vi "Periodic Tasks.vi"(8 "error in":errorcluster) -> ()   [LabVIEW 2017]
doc: "This VI runs in parallel to other tasks. It can contain as many user-defined periodic loops as you need. These can carry out PID or other sorts of timed response."
uses:
  <vilib>/Rock Robotics/WPI/ThirdParty/Phoenix-LabVIEW/Motor Controller/Controls/CTRE_Phoenix_MotorControl_ControlMode.ctl
  <vilib>/Rock Robotics/WPI/ThirdParty/Phoenix-LabVIEW/Motor Controller/Controls/CTRE_Phoenix_MotorControl_LimitSwitchNormal.ctl
  <vilib>/Rock Robotics/WPI/ThirdParty/Phoenix-LabVIEW/Motor Controller/Controls/CTRE_Phoenix_MotorControl_LimitSwitchSource.ctl
  <vilib>/Rock Robotics/WPI/ThirdParty/Phoenix-LabVIEW/Motor Controller/Controls/CTRE_Phoenix_MotorControl_LimitSwitchSource_Local.ctl
  <vilib>/Rock Robotics/WPI/ThirdParty/Phoenix-LabVIEW/Controls/CTRE_Phoenix_Params.ctl
  <vilib>/Rock Robotics/WPI/Utilities/WPI_GetSetVariantRefNum.vi
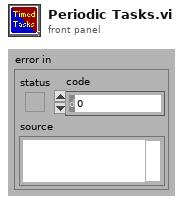
[diagram p1: front panel]
types:
  T1 = typedef "CTRE_CANifier_DeviceRef.ctl" = cluster{"DeviceStatus":errorcluster, "Device Number":u8, "Handle":u64, "UsageFrame":u32, "Library Path":path}
  T2 = typedef "WPI_MotorControlDeviceRef.ctl" = cluster{"DeviceStatus":errorcluster, "Type":T3, "PWM":cluster{"PWM Channel":T4, "DeadBand":T5}, "CAN":cluster{"Device Number":u8, "SetOutput VI Ref":variant, "GetOutput VI Ref":variant, "Enable VI Ref":variant, "Disable VI Ref":variant, "Data":variant}, "Invert":bool, "DIO PWM":cluster{"PWM \"Enable\" Channel":T4, "DIOChannel":T6, "PWM Rate":dbl}}
  T3 = typedef "WPI_MotorControlType.ctl" = enum16{"PWM", "CAN", "DIO PWM"}
  T4 = typedef "FPGA_DIOPWMChannel.ctl" = enum8{"PWM 0", "PWM 1", "PWM 2", "PWM 3", "PWM 4", "PWM 5", "PWM 6", "PWM 7", "PWM 8", "PWM 9", "PWM MXP 0", "PWM MXP 1", "PWM MXP 2", "PWM MXP 3", "PWM MXP 4", "PWM MXP 5", "PWM MXP 6", "PWM MXP 7", "PWM MXP 8", "PWM MXP 9", "Invalid"}
  T5 = typedef "WPI_PWMDeadband.ctl" = cluster{"Name":string, "maxPositivePwm":i32, "minPositivePwm":i32, "centerPwm":i32, "maxNegativePwm":i32, "minNegativePwm":i32, "angularRange":u16}
  T6 = typedef "FPGA_DIOChannel.ctl" = enum8{"DIO 0", "DIO 1", "DIO 2", "DIO 3", "DIO 4", "DIO 5", "DIO 6", "DIO 7", "DIO 8", "DIO 9", "DIO MXP 0", "DIO MXP 1", "DIO MXP 2", "DIO MXP 3", "DIO MXP 4", "DIO MXP 5", "DIO MXP 6", "DIO MXP 7", "DIO MXP 8", "DIO MXP 9", "DIO MXP 10", "DIO MXP 11", "DIO MXP 12", "DIO MXP 13", "DIO MXP 14", "DIO MXP 15", "SPI Port CS1", "SPI Port CS2", "SPI Port CS3", "SPI Port MISO", "SPI Port MOSI", "Invalid"}
  T7 = typedef "WPI_JoystickDevRef.ctl" = cluster{"Device":T8}
  T8 = typedef "WPI_JoystickDeviceEnum.ctl" = enum16{"USB 0", "USB 1", "USB 2", "USB 3", "USB 4", "USB 5"}
  T9 = typedef "CTRE_Phoenix_MotorControl_ControlMode.ctl" = u16
  T10 = typedef "CTRE_Phoenix_MotorControl_LimitSwitchSource.ctl" = u16
  T11 = typedef "CTRE_Phoenix_MotorControl_LimitSwitchNormal.ctl" = enum16{"Normally Open", "Normally Closed", "Disabled"}
  T12 = typedef "CTRE_Phoenix_MotorControl_LimitSwitchSource_Local.ctl" = enum16{"Feedback Connector", "Remote Talon SRX", "Remote CANifier", "Deactivated"}
  T13 = typedef "CTRE_Phoenix_Params.ctl" = u16
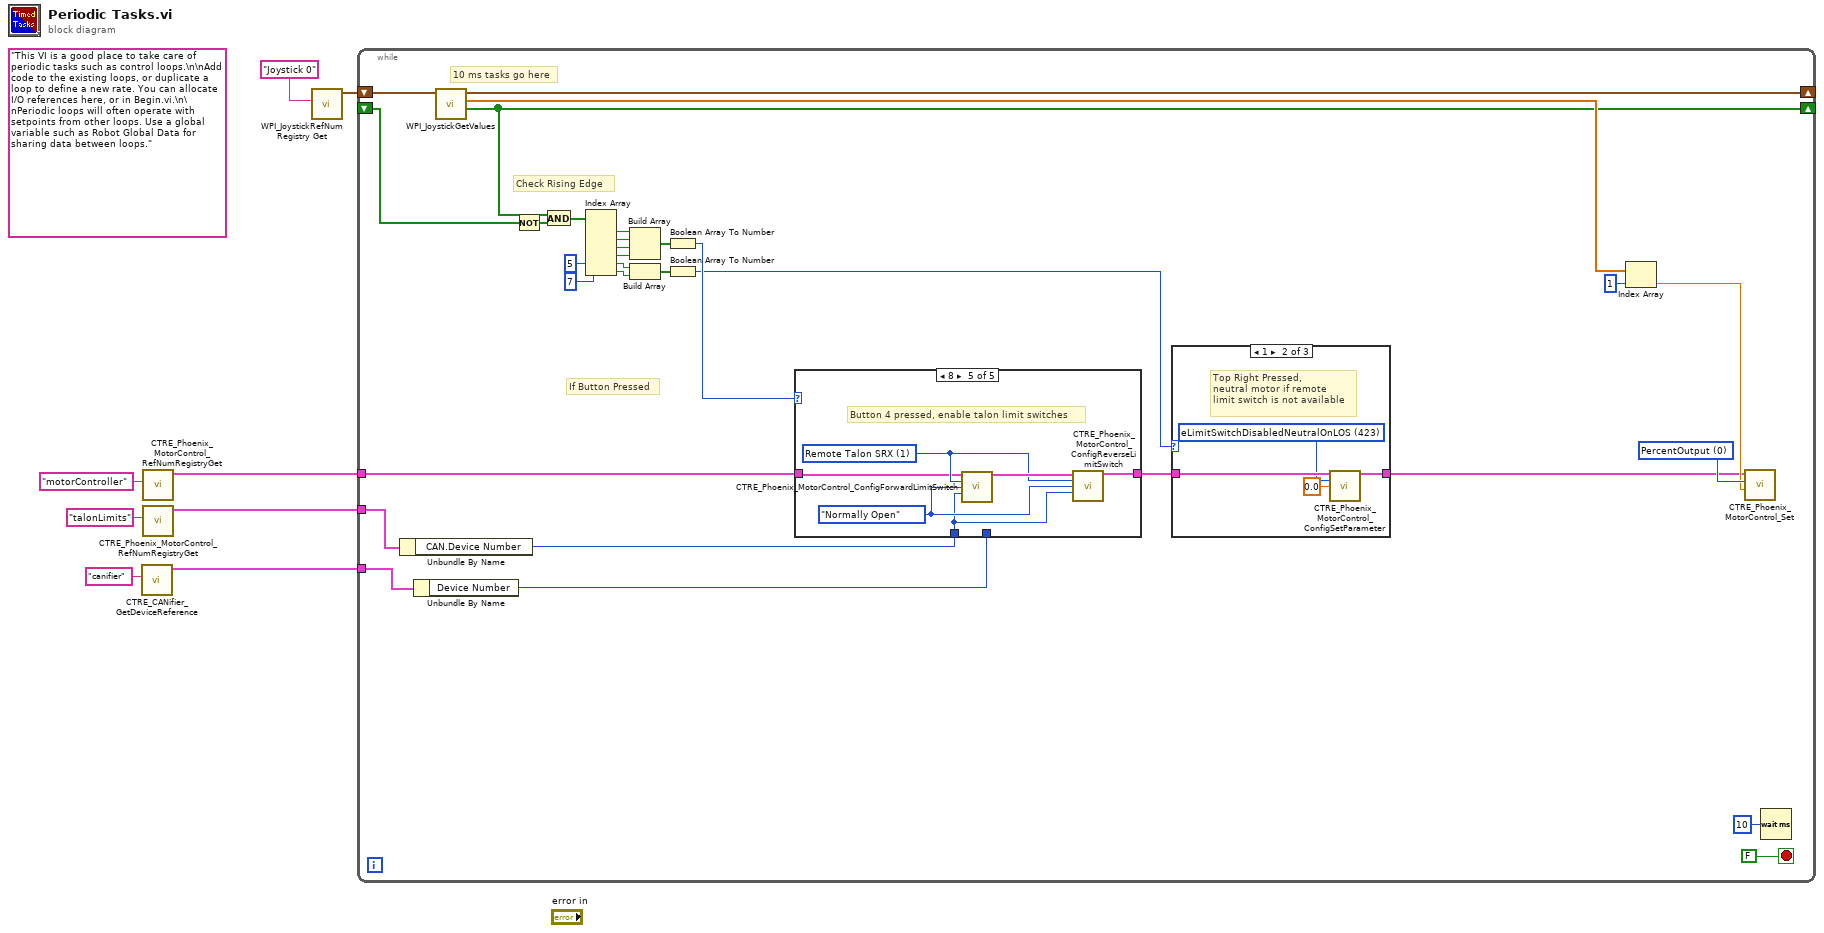
[diagram p0: block diagram]
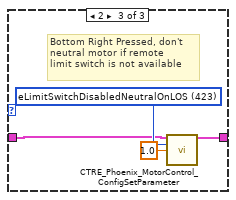
[diagram p3: hidden frame]
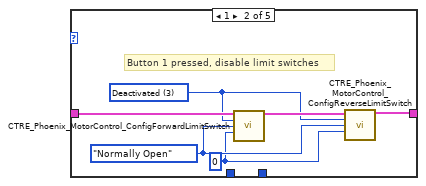
[diagram p5: hidden frame]
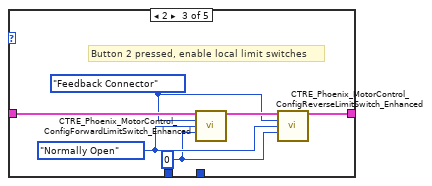
[diagram p6: hidden frame]
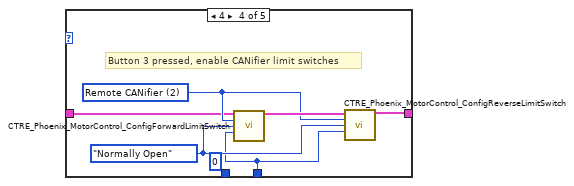
[diagram p7: hidden frame]
diagram:
  (unwired) "This VI is a good place to take care of periodic tasks such as control loops.\n\nAdd code to the existing loops, or duplicate a loop to define a new rate. You can allocate I/O references here, or in Begin.vi.\n\nPeriodic loops will often operate with setpoints from other loops. Use a global variable such as Robot Global Data for sharing data between loops."
  n1 = call <vilib>:"CTRE_CANifier_GetDeviceReference.vi"("refnum name"="canifier") -> ("CANifierDevRef"=w3:T1)  [unwired: 9 in, 1 out]
  n2 = call <vilib>:"CTRE_Phoenix_MotorControl_RefNumRegistryGet.vi"("refnum name"="motorController") -> ("PhoenixMotorControlDevRef"=w1:T2)  [unwired: 9 in, 1 out]
  n3 = call <vilib>:"CTRE_Phoenix_MotorControl_RefNumRegistryGet.vi"("refnum name"="talonLimits") -> ("PhoenixMotorControlDevRef"=w2:T2)  [unwired: 9 in, 1 out]
  n4 = call <vilib>:"WPI_JoystickRefNum Registry Get.vi"("refnum name"="Joystick 0") -> ("JoystickDevRef"=w7:T7)  [unwired: 1 in, 9 out]
  n5 = while {
    shift-right: [w35] -> _
    shift-left: w7 -> [w36]
    tunnel: w3 -> [w23]
    tunnel: w2 -> [w24]
    tunnel: w1 -> [w25]
    shift-right: [w30] -> _
    shift-left: _ -> [w31]
    stop <- FALSE stop-if-true
    w37 = T9 0 items=["PercentOutput"=0, "Position"=1, "Velocity"=2, "Current"=3, "Follower"=5, "MotionProfile"=6, "MotionMagic"=7, "MotionMagicArc"=8, "MotionProfileArc"=10, "Disabled"=15] ("Control Mode")
    # "If Button Pressed"
    # "Check Rising Edge"
    # "10 ms tasks go here"
    n6 = Unbundle By Name(w24) -> ("CAN.Device Number"=w16:u8)
    n7 = Unbundle By Name(w23) -> ("Device Number"=w15:u8)
    n8 = call <vilib>:"WPI_JoystickGetValues.vi"("JoystickDevRef"=w36) -> ("Buttons"=w30:bool[], "Axes"=w34:dbl[], "JoystickDevRef"=w35:T7)  [unwired: 6 in, 2 out]
    n9 = Not(x=w31) -> (.not. x?=w29:bool[])
    n10 = And(x=w30, y=w29) -> (x .and. y?=w26:bool[])
    n11 = Index Array(array=w26, index #5=5 ("index"), index #6=7 ("index")) -> (element #1=w22:bool, element #2=w19:bool, element #3=w20:bool, element #4=w21:bool, element #5=w14:bool, element #6=w13:bool)  [unwired: 4 in]
    n12 = Build Array(w22, w19, w20, w21) -> (w18:bool[])
    n13 = Build Array(w14, w13) -> (w12:bool[])
    n14 = Boolean Array To Number(Boolean array=w18) -> (number=w17:u32)
    n15 = Boolean Array To Number(Boolean array=w12) -> (number=w11:u32)
    n16 = case shown="8" w17 {
      tunnel: w25 -> [w49 w55 w59 w63 w69]
      tunnel: [w49 w53 w60 w62 w70] -> w9
      tunnel: w16 -> [_ _ _ _ w68]
      tunnel: w15 -> [_ _ _ w64 _]
      frame 0, Default {
        # "Nothing pressed"
      }
      frame 1 {
        w52 = T10 3 items=["Remote Talon SRX"=1, "Remote CANifier"=2, "Deactivated"=3] ("LimitSwitchSource")
        w50 = 0 ("deviceID")
        w51 = CTRE_Phoenix_MotorControl_LimitSwitchNormal."Normally Open" ("NormallyOpenOrClosed")
        # "Button 1 pressed, disable limit switches"
        n17 = call <vilib>:"CTRE_Phoenix_MotorControl_ConfigForwardLimitSwitch.vi"("PhoenixMotorControlDevRef"=w55, "LimitSwitchSource"=w52, "NormallyOpenOrClosed"=w51, "deviceID"=w50) -> ("PhoenixMotorControlDevRef"=w54:T2)  [unwired: 10 in, 1 out]
        n18 = call <vilib>:"CTRE_Phoenix_MotorControl_ConfigReverseLimitSwitch.vi"("PhoenixMotorControlDevRef"=w54, "LimitSwitchSource"=w52, "NormallyOpenOrClosed"=w51, "deviceID"=w50) -> ("PhoenixMotorControlDevRef"=w53:T2)  [unwired: 10 in, 1 out]
      }
      frame 2 {
        w56 = 0 ("deviceID")
        w57 = CTRE_Phoenix_MotorControl_LimitSwitchNormal."Normally Open" ("NormallyOpenOrClosed")
        w58 = CTRE_Phoenix_MotorControl_LimitSwitchSource_Local."Feedback Connector" ("Limit Switch Source")
        # "Button 2 pressed, enable local limit switches"
        n19 = call <vilib>:"CTRE_Phoenix_MotorControl_ConfigForwardLimitSwitch_Enhanced.vi"("PhoenixMotorControlDevRef"=w59, "Limit Switch Source"=w58, "NormallyOpenOrClosed"=w57, "deviceID"=w56) -> ("PhoenixMotorControlDevRef"=w61:T2)  [unwired: 10 in, 1 out]
        n20 = call <vilib>:"CTRE_Phoenix_MotorControl_ConfigReverseLimitSwitch_Enhanced.vi"("PhoenixMotorControlDevRef"=w61, "Limit Switch Source"=w58, "NormallyOpenOrClosed"=w57, "deviceID"=w56) -> ("PhoenixMotorControlDevRef"=w60:T2)  [unwired: 10 in, 1 out]
      }
      frame 4 {
        w66 = T10 2 items=["Remote Talon SRX"=1, "Remote CANifier"=2, "Deactivated"=3] ("LimitSwitchSource")
        (unwired) 0 ("deviceID")
        w65 = CTRE_Phoenix_MotorControl_LimitSwitchNormal."Normally Open" ("NormallyOpenOrClosed")
        # "Button 3 pressed, enable CANifier limit switches"
        n21 = call <vilib>:"CTRE_Phoenix_MotorControl_ConfigForwardLimitSwitch.vi"("PhoenixMotorControlDevRef"=w63, "LimitSwitchSource"=w66, "NormallyOpenOrClosed"=w65, "deviceID"=w64) -> ("PhoenixMotorControlDevRef"=w67:T2)  [unwired: 10 in, 1 out]
        n22 = call <vilib>:"CTRE_Phoenix_MotorControl_ConfigReverseLimitSwitch.vi"("PhoenixMotorControlDevRef"=w67, "LimitSwitchSource"=w66, "NormallyOpenOrClosed"=w65, "deviceID"=w64) -> ("PhoenixMotorControlDevRef"=w62:T2)  [unwired: 10 in, 1 out]
      }
      frame 8 {
        w72 = T10 1 items=["Remote Talon SRX"=1, "Remote CANifier"=2, "Deactivated"=3] ("LimitSwitchSource")
        w71 = CTRE_Phoenix_MotorControl_LimitSwitchNormal."Normally Open" ("NormallyOpenOrClosed")
        # "Button 4 pressed, enable talon limit switches"
        n23 = call <vilib>:"CTRE_Phoenix_MotorControl_ConfigForwardLimitSwitch.vi"("PhoenixMotorControlDevRef"=w69, "LimitSwitchSource"=w72, "NormallyOpenOrClosed"=w71, "deviceID"=w68) -> ("PhoenixMotorControlDevRef"=w73:T2)  [unwired: 10 in, 1 out]
        n24 = call <vilib>:"CTRE_Phoenix_MotorControl_ConfigReverseLimitSwitch.vi"("PhoenixMotorControlDevRef"=w73, "LimitSwitchSource"=w72, "NormallyOpenOrClosed"=w71, "deviceID"=w68) -> ("PhoenixMotorControlDevRef"=w70:T2)  [unwired: 10 in, 1 out]
      }
    }
    n25 = case shown="1" w11 {
      tunnel: [w40 w44 w46] -> w10
      tunnel: w9 -> [w40 w43 w45]
      frame 0, Default {
      }
      frame 1 {
        w42 = T13 423 items=["eOnBoot_BrakeMode"=31, "eQuadFilterEn"=91, "eQuadIdxPolarity"=108, "eClearPositionOnIdx"=100, "eMotionProfileHasUnderrunErr"=119, "eMotionProfileTrajectoryPointDurationMs"=120, "eClearPosOnLimitF"=144, "eClearPosOnLimitR"=145, "eStatusFramePeriod"=300, "eOpenLoopRamp"=301, "eClosedLoopRamp"=302, "eNeutralDeadband"=303, "ePeakPosOutput"=305, "eNominalPosOutput"=306, "ePeakNegOutput"=307, "eNominalNegOutput"=308, "eProfileParamSlot_P"=310, "eProfileParamSlot_I"=311, "eProfileParamSlot_D"=312, "eProfileParamSlot_F"=313, "eProfileParamSlot_IZone"=314, "eProfileParamSlot_AllowableErr"=315, "eProfileParamSlot_MaxIAccum"=316, "eClearPositionOnLimitF"=320, "eClearPositionOnLimitR"=321, "eClearPositionOnQuadIdx"=322, "eSampleVelocityPeriod"=325, "eSampleVelocityWindow"=326, "eFeedbackSensorType"=330, "eSelectedSensorPosition"=331, "eFeedbackNotContinuous"=332, "eRemoteSensorSource"=333, "eRemoteSensorDeviceID"=334, "eSensorTerm"=335, "eRemoteSensorClosedLoopDisableNeutralOnLOS"=336, "eForwardSoftLimitThreshold"=340, "eReverseSoftLimitThreshold"=341, "eForwardSoftLimitEnable"=342, "eReverseSoftLimitEnable"=343, "eNominalBatteryVoltage"=350, "eBatterVoltageFilterSize"=351, "eContinuousCurrentLimitAmps"=360, "eContinuousCurrentLimitMs"=361, "ePeakCurrentLimitAmps"=362, "eClosedLoopIAccum"=370, "eCustomParam"=380, "eStickyFaults"=390, "eAnalogPosition"=400, "eQuadraturePosition"=401, "ePulseWidthPosition"=402, "eMotMag_Accel"=410, "eMotMag_VelCruise"=411, "eLimitSwitchSource"=421, "eLimitSwitchNormClosedAndDis"=422, "eLimitSwitchDisabledNeutralOnLOS"=423, "eLimitSwitchRemoteDevID"=424] ("Parameter")
        # "Top Right Pressed,\nneutral motor if remote\nlimit switch is not available"
        n26 = call <vilib>:"CTRE_Phoenix_MotorControl_ConfigSetParameter.vi"("PhoenixMotorControlDevRef"=w43, "Parameter"=w42, "value"=0.0) -> ("PhoenixMotorControlDevRef"=w44:T2)  [unwired: 11 in, 1 out]
      }
      frame 2 {
        w48 = T13 423 items=["eOnBoot_BrakeMode"=31, "eQuadFilterEn"=91, "eQuadIdxPolarity"=108, "eClearPositionOnIdx"=100, "eMotionProfileHasUnderrunErr"=119, "eMotionProfileTrajectoryPointDurationMs"=120, "eClearPosOnLimitF"=144, "eClearPosOnLimitR"=145, "eStatusFramePeriod"=300, "eOpenLoopRamp"=301, "eClosedLoopRamp"=302, "eNeutralDeadband"=303, "ePeakPosOutput"=305, "eNominalPosOutput"=306, "ePeakNegOutput"=307, "eNominalNegOutput"=308, "eProfileParamSlot_P"=310, "eProfileParamSlot_I"=311, "eProfileParamSlot_D"=312, "eProfileParamSlot_F"=313, "eProfileParamSlot_IZone"=314, "eProfileParamSlot_AllowableErr"=315, "eProfileParamSlot_MaxIAccum"=316, "eClearPositionOnLimitF"=320, "eClearPositionOnLimitR"=321, "eClearPositionOnQuadIdx"=322, "eSampleVelocityPeriod"=325, "eSampleVelocityWindow"=326, "eFeedbackSensorType"=330, "eSelectedSensorPosition"=331, "eFeedbackNotContinuous"=332, "eRemoteSensorSource"=333, "eRemoteSensorDeviceID"=334, "eSensorTerm"=335, "eRemoteSensorClosedLoopDisableNeutralOnLOS"=336, "eForwardSoftLimitThreshold"=340, "eReverseSoftLimitThreshold"=341, "eForwardSoftLimitEnable"=342, "eReverseSoftLimitEnable"=343, "eNominalBatteryVoltage"=350, "eBatterVoltageFilterSize"=351, "eContinuousCurrentLimitAmps"=360, "eContinuousCurrentLimitMs"=361, "ePeakCurrentLimitAmps"=362, "eClosedLoopIAccum"=370, "eCustomParam"=380, "eStickyFaults"=390, "eAnalogPosition"=400, "eQuadraturePosition"=401, "ePulseWidthPosition"=402, "eMotMag_Accel"=410, "eMotMag_VelCruise"=411, "eLimitSwitchSource"=421, "eLimitSwitchNormClosedAndDis"=422, "eLimitSwitchDisabledNeutralOnLOS"=423, "eLimitSwitchRemoteDevID"=424] ("Parameter")
        # "Bottom Right Pressed, don't\nneutral motor if remote\nlimit switch is not available"
        n27 = call <vilib>:"CTRE_Phoenix_MotorControl_ConfigSetParameter.vi"("PhoenixMotorControlDevRef"=w45, "Parameter"=w48, "value"=1.0) -> ("PhoenixMotorControlDevRef"=w46:T2)  [unwired: 11 in, 1 out]
      }
    }
    n28 = Index Array(array=w34, index=1) -> (element=w32:dbl)
    n29 = call <vilib>:"CTRE_Phoenix_MotorControl_Set.vi"("Output"=w32, "Control Mode"=w37, "PhoenixMotorControlDevRef"=w10) -> ()  [unwired: 7 in, 2 out]
    n30 = Wait (ms)(milliseconds to wait=u32 10) -> ()  [unwired: 1 out]
  }
